vi "createReportServerStatusFrame.vi"(8 "error in (no error)":errorcluster, 9 "TriggerIRQ":bool, 10 "WaitForTrigger":bool, 11 "ILC in":refnum<class "ILC.lvclass">) -> (0 "error out":errorcluster, 2 "TxFrame":T1 {"Data" format="%02x"}, 3 "ILC out":refnum<class "ILC.lvclass">)   [LabVIEW 2016, in "RTILC.lvlib" / "ILC.lvclass"]
uses:
  ILC.lvclass
  Common_RT_Modbus/DataTypes/TxFrame.ctl
  Common_RT_Modbus/DynamicFrameBuilder/DynamicFrameBuilder.lvclass
  ILC.lvclass/ILC.ctl
  Common_RT_Modbus/RTModbus.lvlib
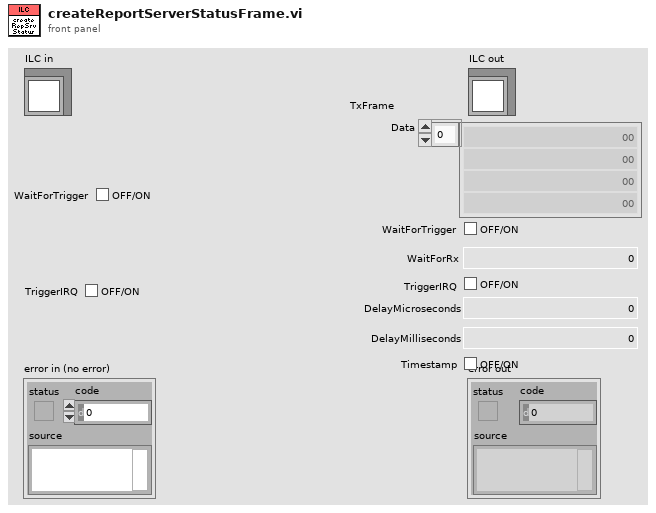
[diagram p1: front panel]
types:
  T1 = typedef "RTModbus.lvlib/TxFrame.ctl" = cluster{"Data":u8[], "WaitForTrigger":bool, "WaitForRx":u16, "TriggerIRQ":bool, "DelayMicroseconds":u16, "DelayMilliseconds":u16, "Timestamp":bool}
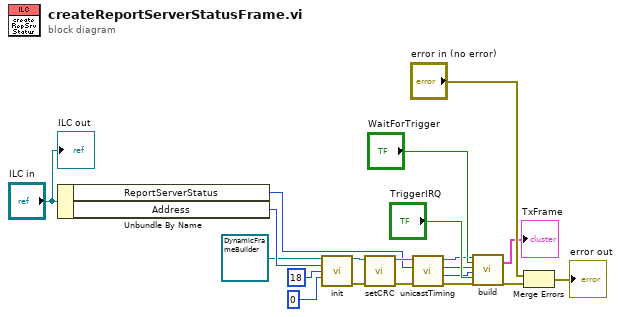
[diagram p0: block diagram]
diagram:
  n1 = Unbundle By Name("ILC in") -> ("ReportServerStatus"=w5:u32, "Address"=w17:u8)
  n2 = call "init.vi"("DynamicFrameBuilder in"=refnum<class "DynamicFrameBuilder.lvclass"> refnum ("RTModbus.lvlib:DynamicFrameBuilder.lvclass"), "Address"=w17, "Function"=u8 18, "DataSize"=0) -> ("DynamicFrameBuilder out"=w13:refnum<class "DynamicFrameBuilder.lvclass">, "error out"=w11:errorcluster)  [unwired: 10 in]
  n3 = call "setCRC.vi"("error in (no error)"=w11, "DynamicFrameBuilder in"=w13) -> ("error out"=w6:errorcluster, "DynamicFrameBuilder out"=w7:refnum<class "DynamicFrameBuilder.lvclass">)  [unwired: 8 in]
  n4 = call "unicastTiming.vi"("error in (no error)"=w6, "Latency in"=w5, "DynamicFrameBuilder in"=w7) -> ("error out"=w2:errorcluster, "WaitForRxTimeout"=w3:u16, "Latency out"=w4:u32, "DynamicFrameBuilder out"=w1:refnum<class "DynamicFrameBuilder.lvclass">)  [unwired: 5 in]
  n5 = call "build.vi"("DynamicFrameBuilder in"=w1, "WaitForTrigger"="WaitForTrigger", "Latency"=w4, "WaitForRxTimeout"=w3, "TriggerIRQ"="TriggerIRQ", "error in (no error)"=w2) -> ("TxFrame"=→"TxFrame":T1, "error out"=w10:errorcluster)  [unwired: 11 in, 1 out]
  n6 = Merge Errors("error in (no error)", w10) -> (→"error out":errorcluster)
  "ILC out" <- "ILC in"
